vi "ForwardKinematics.vi"(9 "dHeading (rad)":dbl(slide) step=0.001 scale=-1.0..1.0, 11 "dX":dbl(slide) scale=0.0..10.0) -> (1 "dY":dbl, 3 "dX":dbl)   [LabVIEW 2018]
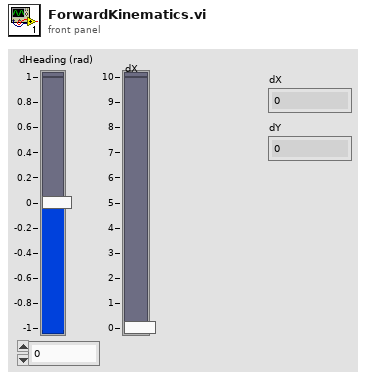
[diagram p1: front panel]
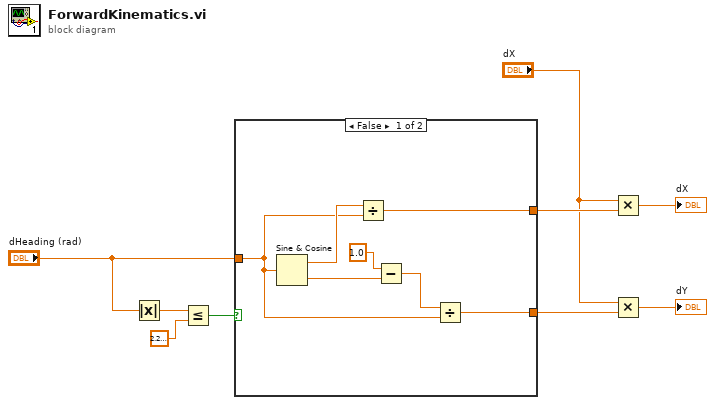
[diagram p0: block diagram]
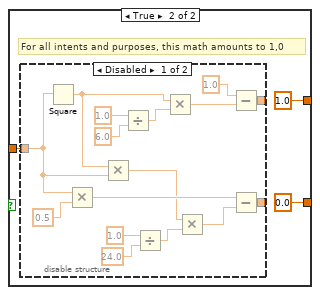
[diagram p2: hidden frame]
diagram:
  n1 = Absolute Value(x="dHeading (rad)") -> (abs(x)=w9:dbl)
  n2 = Less Or Equal?(x=w9, y=2.220446049250313e-16) -> (x <= y?=w7:bool)
  n3 = case shown="False" w7 {
    tunnel: [w11 1.0] -> w5
    tunnel: [w12 0.0] -> w4
    tunnel: "dHeading (rad)" -> [w10 w17]
    frame False {
      n4 = Sine & Cosine(0:w10) -> (1:w16:dbl, 2:w15:dbl)
      n5 = Divide(x=w16, y=w10) -> (x/y=w11:dbl)
      n6 = Subtract(x=1.0, y=w15) -> (x-y=w13:dbl)
      n7 = Divide(x=w13, y=w10) -> (x/y=w12:dbl)
    }
    frame True {
      # "For all intents and purposes, this math amounts to 1,0"
      n8 = disable-structure shown="Disabled" {
        disable-tunnel: [w29 _] -> _
        disable-tunnel: [w27 _] -> _
        disable-tunnel: w17 -> [w22 _]
        frame Disabled {
          n9 = Square(x=w22) -> (x^2=w23:dbl)
          n10 = Multiply(x=w22, y=0.5) -> (x*y=w28:dbl)
          n11 = Multiply(x=w23, y=w22) -> (x*y=w21:dbl)
          n12 = Divide(x=1.0, y=6.0) -> (x/y=w31:dbl)
          n13 = Divide(x=1.0, y=24.0) -> (x/y=w24:dbl)
          n14 = Multiply(x=w23, y=w31) -> (x*y=w30:dbl)
          n15 = Multiply(x=w21, y=w24) -> (x*y=w20:dbl)
          n16 = Subtract(x=1.0, y=w30) -> (x-y=w29:dbl)
          n17 = Subtract(x=w28, y=w20) -> (x-y=w27:dbl)
        }
        frame Enabled {
        }
      }
    }
  }
  n18 = Multiply(x="dX", y=w5) -> (x*y=→"dX":dbl)
  n19 = Multiply(x="dX", y=w4) -> (x*y=→"dY":dbl)
